vi "Status Acquisition.vi"(4 "error in (no error)":errorcluster, 7 "status":i32) -> (0 "error out":errorcluster, 2 "function return":i32, 3 "status out":i32)   [LabVIEW 2020, in "ThorConfocal.lvlib"]
doc: "long StatusAcquisition(long &status);"
uses:
  ThorConfocal.lvlib
  ThorConfocal.dll
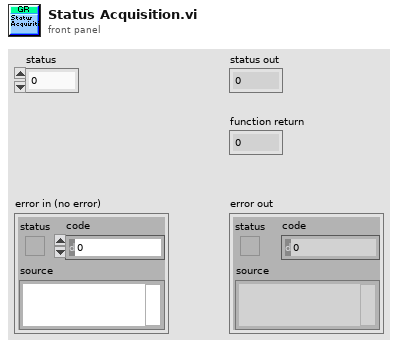
[diagram p1: front panel]
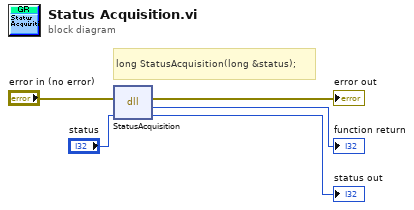
[diagram p0: block diagram]
diagram:
  # "long StatusAcquisition(long &status);"
  n1 = dll-call lib="D:/software/TweezerTron/ThorConfocal.dll" fn="StatusAcquisition"(error in="error in (no error)", "status"="status") -> (error out=→"error out":errorcluster, "return type"=→"function return":i32, "status"=→"status out":i32)  [unwired: 2 in, 1 out]
